vi "Engine Knocking Monitor.vi"() -> ()   [LabVIEW 2023]
doc: "This example shows the application of autoregressive-moving average (ARMA) modeling in examining the condition of an engine.\n\nUnder normal conditions, the vibration signal from the engine is a stationary time series. If you build an ARMA model for the stationary time series, the modeling errors are usually small. However, if the engine is not running properly due to imbalance or cracks, the vibration signal becomes a nonstationary time series. If you build an ARMA model for this nonstationary time series, the modeling errors increase. \n\nThis example uses the TSA ARMA Modeling VI to build an ARMA model for the vibration signal of an engine and uses the TSA Deviation and Variation VI to compute the noise variances, or errors, of the modeling.\n\n<b>Instructions:</b>\n1) Run this VI.\n2) Set the threshold for the noise variance. When the noise variance is greater than the threshold, Fault mode? becomes TRUE."
uses:
  <vilib>/addons/Time Series Analysis/Utilities.llb/TSA Data.ctl
  <vilib>/addons/Time Series Analysis/Modeling and Prediction.llb/TSA ARMA Modeling (Waveform).vi
  <vilib>/addons/Time Series Analysis/Statistical Analysis.llb/TSA Deviation and Variance (Waveform).vi
  <vilib>/addons/_Advanced Signal Processing/NI_AdvSigProcTSA.lvlib
panel:
  in  "Threshold":dbl(slide) scale=0.0..30000000.0
  out "Fault Mode?":bool
  in  "stop":bool
  out "Vibration Series":waveform(dbl)(graph)
  out "Noise Variance":cluster{"variance":dbl, "Threshold":dbl}(graph)
  # "Overview: Shows the application of autoregressive-moving average (ARMA) modeling in examining the condition of an engine.\nRequirements: LabVIEW Full Development System, Advanced Signal Processing Toolkit\nInstructions: \n1. Run this VI.\n2. Set the threshold for the noise variance. When the noise variance is greater than the threshold, Fault mode? returns TRUE.\n3. Click Stop to stop the VI."
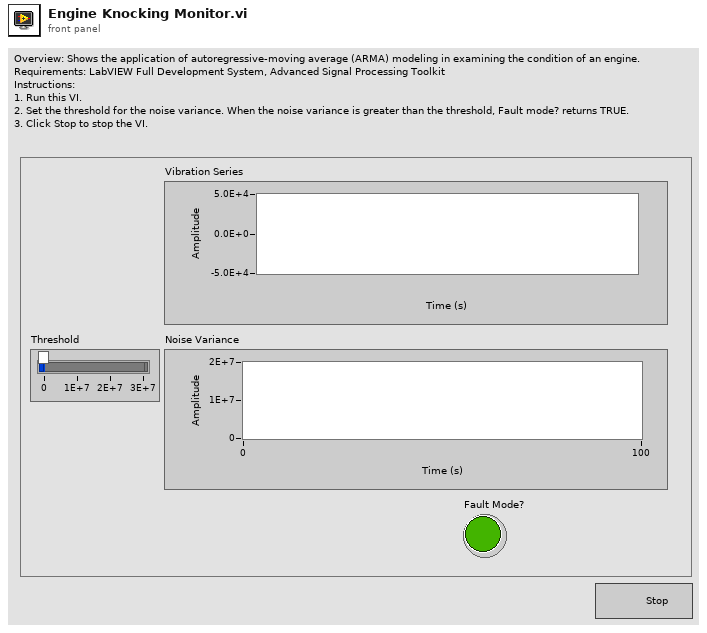
[diagram p1: front panel]
types:
  T1 = typedef "NI_AdvSigProcTSA.lvlib/TSA Data.ctl" = u16
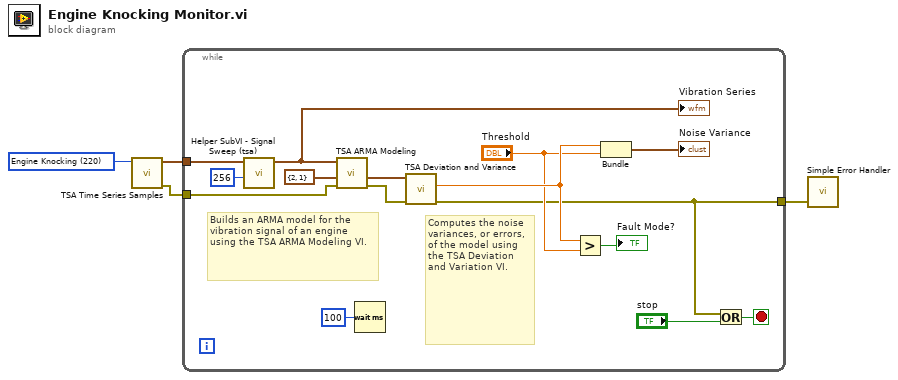
[diagram p0: block diagram]
diagram:
  w3 = T1 220 items=["Kobe Earthquake"=201, "EEG"=210, "Bearing Vibration (simulated)"=211, "Period Product Sales"=214, "Beam Vibration (nonlinear)"=217, "Beam Vibration (linear)"=218, "Signal With Echo"=219, "Engine Knocking"=220, "Power Line"=221, "-"=200, "Beam Deflections (multivariate)"=207, "Structure Vibration (multivariate)"=208, "Human MEG (multivariate)"=222] ("data")
  n1 = call <vilib>:"TSA Time Series Samples.vi"("data"=w3) -> ("error out"=w1:errorcluster, "univariate time series"=w4:waveform(dbl))  [unwired: 1 in, 8 out]
  n2 = while {
    tunnel: w4 -> [w12]
    tunnel: [w6] -> w2
    tunnel: w1 -> [w5]
    stop <- w7 stop-if-true
    # "Computes the noise variances, or errors, of the model using the TSA Deviation and Variation VI."
    # "Builds an ARMA model for the vibration signal of an engine\nusing the TSA ARMA Modeling VI."
    n3 = call "Helper SubVI - Signal Sweep (tsa).vi"("length"=256, "Signal in"=w12) -> ("Signal out"=w10:waveform(dbl))  [unwired: 9 in]
    "Vibration Series" <- w10
    n4 = call-poly <vilib>:"TSA ARMA Modeling.vi"("error in (no error)"=w5, "ARMA order"=cluster{"AR":i32, "MA":i32} {"AR"=2, "MA"=1}, "Xt"=w10) -> ("error out"=w9:errorcluster, "noise"=w16:waveform(dbl))  [unwired: 1 in, 6 out]
    n5 = Wait (ms)(milliseconds to wait=u32 100 ("millisecond multiple")) -> ()  [unwired: 1 out]
    n6 = call-poly <vilib>:"TSA Deviation and Variance.vi"("error in (no error)"=w9, "Xt"=w16) -> ("error out"=w6:errorcluster, "variance"=w17:dbl)  [unwired: 1 in, 7 out]
    n7 = Greater?(x=w17, y="Threshold") -> (0:→"Fault Mode?":bool)
    n8 = Bundle("variance"=w17, "Threshold"="Threshold") -> (→"Noise Variance":cluster{"variance":dbl, "Threshold":dbl})  [unwired: 1 out]
    n9 = Or(x=w6, y="stop") -> (x .or. y?=w7:bool)
  }
  n10 = call <vilib>:"Simple Error Handler.vi"("error in (no error)"=w2) -> ()  [unwired: 4 in, 5 out]
